vi "InjectModel.vi"(8 "error in (no error)":errorcluster, 10 "Model":refnum<class "Model.lvclass">, 11 "View in":refnum<class "View.lvclass">) -> (0 "error out":errorcluster, 3 "View out":refnum<class "View.lvclass">)   [LabVIEW 2020, in "Page1.lvlib" / "View.lvclass"]
uses:
  View.lvclass
  Model/Model/Model.lvclass
  View.lvclass/View.ctl
  Controller/Controller.lvclass
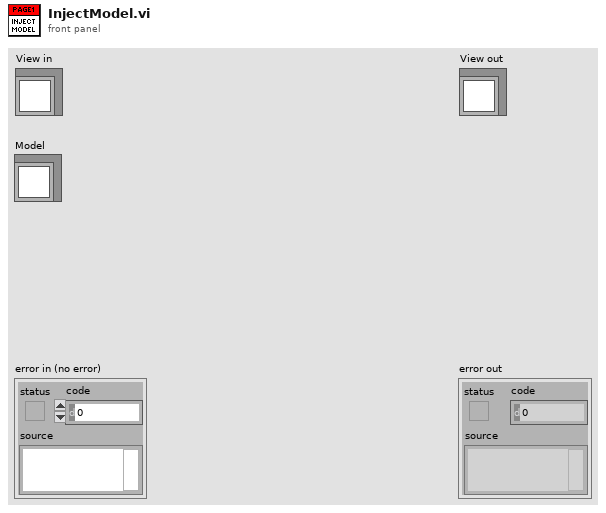
[diagram p1: front panel]
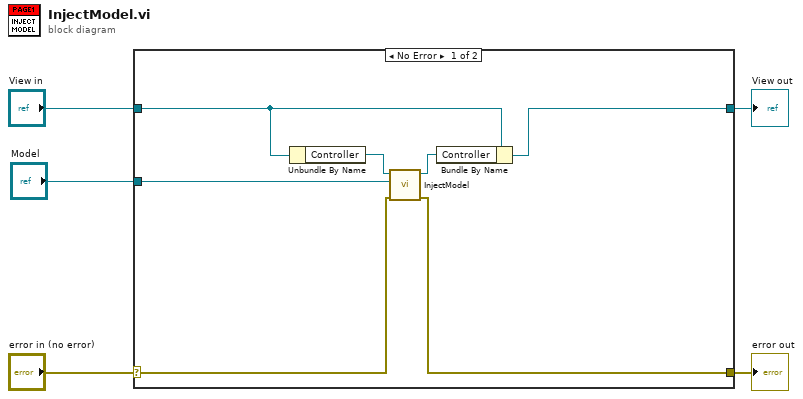
[diagram p0: block diagram]
diagram:
  n1 = case shown="No Error" "error in (no error)" {
    selector: "error in (no error)" -> [w10 w14]
    tunnel: [w6 w14] -> w4
    tunnel: [w7 w13] -> w2
    tunnel: "View in" -> [w9 w13]
    tunnel: "Model" -> [w11 _]
    frame No Error {
      n2 = Unbundle By Name(w9) -> ("Controller"=w12:refnum<class "Controller.lvclass">)
      n3 = call "InjectModel.vi"("error in (no error)"=w10, "Model"=w11, "Controller in"=w12) -> ("error out"=w6:errorcluster, "Controller out"=w8:refnum<class "Controller.lvclass">)  [unwired: 7 in]
      n4 = Bundle By Name(cluster=w9, "Controller"=w8) -> (w7:refnum<class "View.lvclass">)
    }
    frame Error {
    }
  }
  "error out" <- w4
  "View out" <- w2
